vi "FGV_Current Device.vi"(8 "error in (no error)":errorcluster caption="错误输入（无错误）", 10 "Set":bool, 11 "CurrentDev":T1={"Type"=41, "Index"=0} {"Index" items=["0", "1", "2", "3", "4", "5", "6", "7", "8"]; "Type" items=["USBCANFD-200U"=41, "USBCANFD-100U"=42]}) -> (0 "error out":errorcluster caption="错误输出", 3 "CurrentDev out":T1={"Type"=41, "Index"=0} {"Index" items=["0", "1", "2", "3", "4", "5", "6", "7", "8"]; "Type" items=["USBCANFD-200U"=41, "USBCANFD-100U"=42]})   [LabVIEW 2018, in "CAN FD.lvlib"]
uses:
  CAN FD.lvlib
  Typedef/CurrentDev.ctl
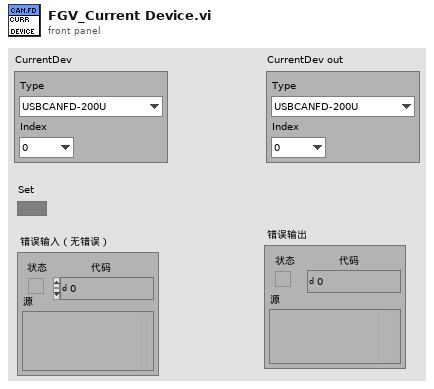
[diagram p1: front panel]
types:
  T1 = typedef "CAN FD.lvlib/CurrentDev.ctl" = cluster{"Type":u32, "Index":u32}
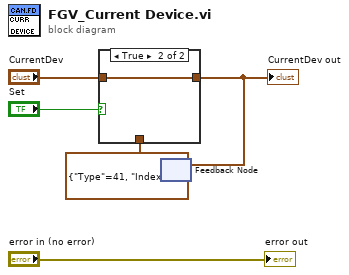
[diagram p0: block diagram]
diagram:
  n1 = feedback #1(T1 {"Type"=41, "Index"=0} ("CurrentDev")) -> (w2:T1)
  n2 = case shown="True" "Set" {
    tunnel: [w7 w8] -> w3
    tunnel: "CurrentDev" -> [_ w8]
    tunnel: w2 -> [w7 _]
    frame False {
    }
    frame True {
    }
  }
  "CurrentDev out" <- w3
  n3 = feedback-in #1(w3) -> ()
  "error out" <- "error in (no error)"
